vi "Test 6.vi"(8 "error in (no error)":errorcluster, 11 "Test Case In":refnum<class "Tests.lvclass">) -> (0 "error out":errorcluster, 3 "Test Case Out":refnum<class "Tests.lvclass">)   [LabVIEW 2020, in "Tests.lvclass"]
uses:
  Tests.lvclass
  C:/Program Files (x86)/National Instruments/LabVIEW 2020/vi.lib/Astemes/LUnit/Test Case.lvclass
  <vilib>/Astemes/LUnit/Test Case.lvclass/Test Case.ctl
  4993e8ee-a06a-463a-9684-69129f64d5ce.vi
  <vilib>/Astemes/LUnit/Append Pass Result.vi
  <vilib>/Astemes/LUnit/Append Fail Result.vi
  <vilib>/Astemes/LUnit/Describe Comparison.vi
  4993e8ee-a06a-463a-9684-69129f64d5ce.vi/9c5d11cd-9439-4240-a1ee-d9baace9c924.vi
  <vilib>/Astemes/LUnit/Run In UI.vi
  <vilib>/Utility/error.llb/Clear Errors.vi
  <vilib>/Astemes/LUnit/Describe Variant.vi
  Proto/NetAn.lvclass
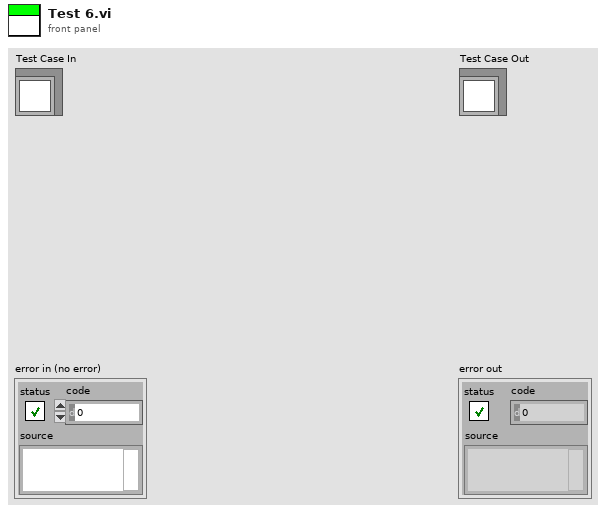
[diagram p1: front panel]
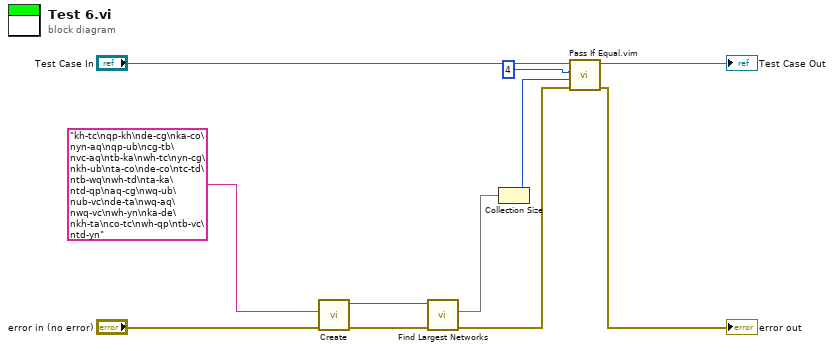
[diagram p0: block diagram]
diagram:
  n1 = call "Create.vi"("error in (no error)"="error in (no error)", "Input"="kh-tc\nqp-kh\nde-cg\nka-co\nyn-aq\nqp-ub\ncg-tb\nvc-aq\ntb-ka\nwh-tc\nyn-cg\nkh-ub\nta-co\nde-co\ntc-td\ntb-wq\nwh-td\nta-ka\ntd-qp\naq-cg\nwq-ub\nub-vc\nde-ta\nwq-aq\nwq-vc\nwh-yn\nka-de\nkh-ta\nco-tc\nwh-qp\ntb-vc\ntd-yn") -> ("error out"=w8:errorcluster, "Proto"=w5:refnum<class "NetAn.lvclass">)  [unwired: 8 in]
  n2 = call "Find Largest Networks.vi"("error in (no error)"=w8, "Proto in"=w5) -> ("error out"=w6:errorcluster, "set"=w4:set{string})  [unwired: 7 in, 1 out]
  n3 = Collection Size(1:w4) -> (0:w3:i32)
  n4 = call "Pass If Equal.vim"("error in (no error)"=w6, "Actual"=w3, "Expected"=4, "LUnit Test Case In"="Test Case In") -> ("error out"=→"error out":errorcluster, "LUnit Test Case Out"=→"Test Case Out":refnum<class "Tests.lvclass">)  [unwired: 6 in]
